vi "SMC TestProgram.vi"() -> ()   [LabVIEW 2015]
uses:
  SubVIs/JS_Misc.llb/JS_Axis_PM.ctl
  SubVIs/JS_Comm.llb/Comm_Paras.ctl
  SubVIs/JS_Comm.llb/Comm_Method.ctl
  SMC SubVIs/SMC_SubVIs.llb/SMC Paras.ctl
  SMC SubVIs/SMC_SubVIs.llb/VENUSNr.ctl
  SMC SubVIs/SMC_SubVIs.llb/glb_stop.vi
  SMC SubVIs/SMC_SubVIs.llb/glb_pos.vi
panel:
  in  "Show Dialog Box":bool=TRUE
  in  "Error":bool
  in  "Controller Nr":u8=3 min=1 max=10 step=1
  out "Communication":bool
  out "Communication Error":bool
  out "Position":dbl[](array[numeric]) format="%.6f"
  out "Moving":bool
  in  "Stop":bool
  in  "Tab Control":enum32{"Standard", "low level"}(tab)
  in  "Velocity":bool
  in  "Move absolute":bool
  in  "Destination [mm]":dbl[](array[numeric]) format="%.6f"
  in  "Manual Control":T1[](array[typedef])
  in  "RefMove":bool
  in  "SetZero":bool
  in  "StepWidth [mm]":dbl=1.0 format="%.6f"
  in  "RangeMeasure":bool
  in  "Calibrate":bool
  in  "Switch Status":bool
  in  "Limit":bool
  in  "Maeander":bool
  in  "Sequence":bool
  in  "Get Error":bool
  out "ErrorText":string
  out "Error Code":string
  out "Result":string
  in  "Command":string
  in  "Send":bool
  out "End Prog":bool
  out "error out":errorcluster
  in  "End Program":bool
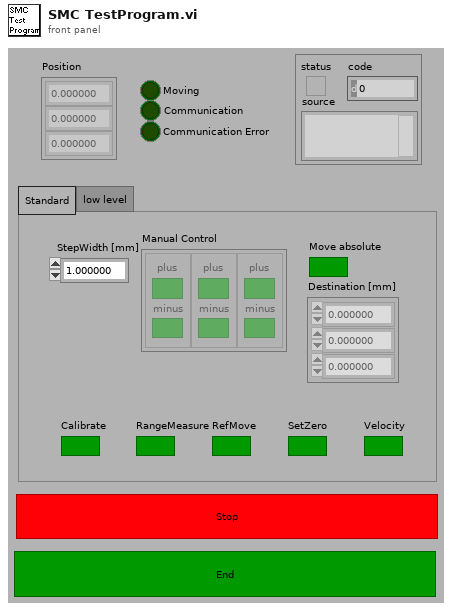
[diagram p1: front panel]
types:
  T1 = typedef "JS_Axis_PM.ctl" = cluster{"minus":bool, "plus":bool}
  T2 = typedef "SMC Paras.ctl" = cluster{"VENUS Language":T3, "Number of Axis":u8, "Controller Nr":u8, "Simulation":bool}
  T3 = typedef "VENUSNr.ctl" = enum16{"VENUS 2", "VENUS 1"}
  T4 = typedef "Comm_Paras.ctl" = cluster{"Comm Method":T5, "Com Port":i32, "Baud Rate":u32, "IP Address":string, "Remote Port":u16, "GPIB Address":string, "VISA Resource Name":refnum<visa-resource-name>, "Visa Baud Rate":u32, "Visa Serial":bool}
  T5 = typedef "Comm_Method.ctl" = enum16{"RS232", "TCPIP", "GPIB", "VISA"}
  T6 = typedef "Sequence Paras.ctl" = cluster{"Number of cycles":i32, "Start position":dbl[], "End position":dbl[]}
  T7 = typedef "Maeander_Paras.ctl" = cluster{"Number":i32, "X Start":dbl, "Y Start":dbl, "X Size":dbl, "Y Size":dbl}
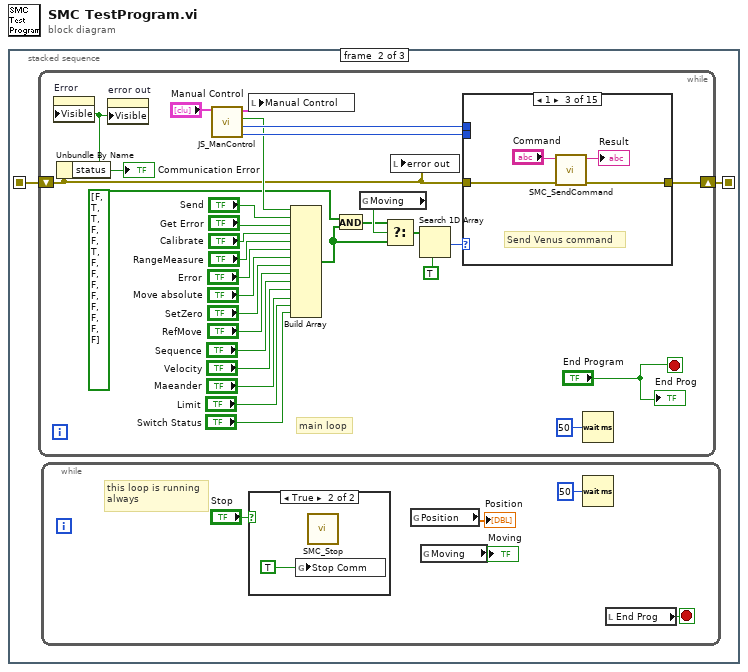
[diagram p0: block diagram]
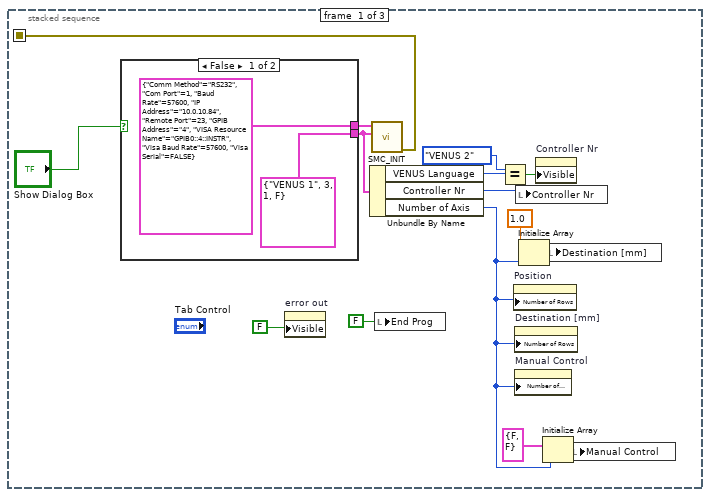
[diagram p2: hidden frame]
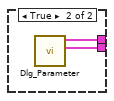
[diagram p3: hidden frame]
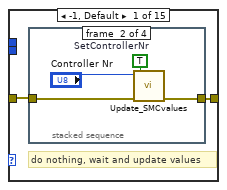
[diagram p5: hidden frame]
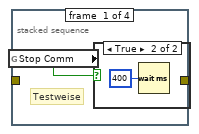
[diagram p6: hidden frame]
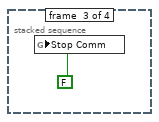
[diagram p8: hidden frame]
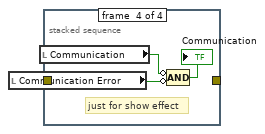
[diagram p9: hidden frame]
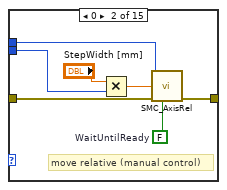
[diagram p10: hidden frame]
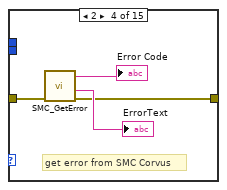
[diagram p11: hidden frame]
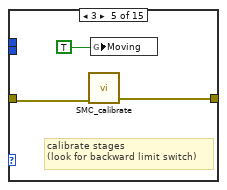
[diagram p12: hidden frame]
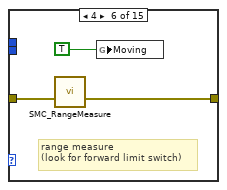
[diagram p13: hidden frame]
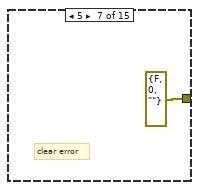
[diagram p14: hidden frame]
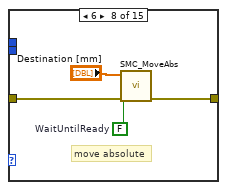
[diagram p15: hidden frame]
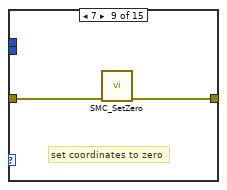
[diagram p16: hidden frame]
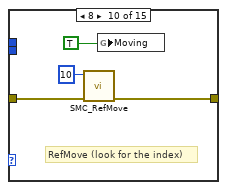
[diagram p17: hidden frame]
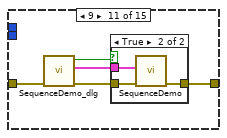
[diagram p18: hidden frame]
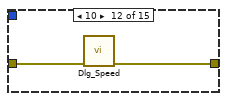
[diagram p20: hidden frame]
diagram:
  n1 = stacked-sequence {
    seq-local: [w11 _ _] -> [_ w21 _]
    seq-local: [_ w20 _] -> [_ _ w128]
    frame #0 {
      n2 = case shown="False" "Show Dialog Box" {
        tunnel: [T4 {"Comm Method"=enum."RS232", "Com Port"=1, "Baud Rate"=57600, "IP Address"="10.0.10.84", "Remote Port"=23, "GPIB Address"="4", "VISA Resource Name"="GPIB0::4::INSTR", "Visa Baud Rate"=57600, "Visa Serial"=FALSE} ("Communication Parameter") w19] -> w9
        tunnel: [T2 {"VENUS Language"=enum."VENUS 1", "Number of Axis"=3, "Controller Nr"=1, "Simulation"=FALSE} ("SMC Parameter") w18] -> w7
        frame False {
        }
        frame True {
          n3 = call "Dlg_Parameter.vi"() -> ("SMC Parameter"=w18:T2, "Communication Parameter"=w19:T4)  [unwired: 10 in]
        }
      }
      n4 = property on="error out" class="Clust (strict)"("Visible"=FALSE ("Write Attribute")) -> ()  [unwired: 2 in, 2 out]
      n5 = Unbundle By Name(w7) -> ("VENUS Language"=w6:T3, "Controller Nr"=w4:u8, "Number of Axis"=w2:u8)
      n6 = call "SMC_INIT.vi"("SMC Parameter"=w7, "Communication Parameter"=w9) -> ("error out"=w11:errorcluster)  [unwired: 9 in]
      n7 = local write "End Prog"(FALSE ("End Prog")) -> ()
      n8 = Equal?(x=enum16{"VENUS 2", "VENUS 1"}."VENUS 2" ("y"), y=w6) -> (x = y?=w8:bool)
      n9 = property on="Position" class="Arr (strict)"("Number of Rows"=w2) -> ()  [unwired: 2 in, 2 out]
      n10 = property on="Destination [mm]" class="Arr (strict)"("Number of Rows"=w2) -> ()  [unwired: 2 in, 2 out]
      n11 = property on="Manual Control" class="Arr"("Number of Columns"=w2) -> ()  [unwired: 2 in, 2 out]
      n12 = local write "Controller Nr"(w4) -> ()
      n13 = Initialize Array(1.0, w2) -> (w12:dbl[])
      n14 = property on="Controller Nr" class="DigNum (strict)"("Visible"=w8) -> ()  [unwired: 2 in, 2 out]
      n15 = Initialize Array(T1 {"minus"=FALSE, "plus"=FALSE} ("Cluster"), w2) -> (w1:T1[])
      n16 = local write "Destination [mm]"(w12) -> ()
      n17 = local write "Manual Control"(w1) -> ()
    }
    frame #1 {
      n18 = while {
        shift-right: [w30] -> w20
        shift-left: w21 -> [w28]
        stop <- "End Program" stop-if-true
        # "main loop"
        n19 = Unbundle By Name(w28) -> ("status"=w29:bool)
        "Communication Error" <- w29
        n20 = property on="Error" class="Bool"("Visible"=w29) -> ()  [unwired: 2 in, 2 out]
        n21 = property on="error out" class="Clust (strict)"("Visible"=w29) -> ()  [unwired: 2 in, 2 out]
        n22 = call "JS_ManControl.vi"("Manual Control in"="Manual Control") -> ("Manual Control out"=w47:T1[], "Fire"=w45:bool, "AxisNr"=w48:i32, "sign"=w46:i8)
        n23 = local write "Manual Control"(w47) -> ()
        n24 = Build Array(w45, "Send", "Get Error", "Calibrate", "RangeMeasure", "Error", "Move absolute", "SetZero", "RefMove", "Sequence", "Velocity", "Maeander", "Limit", "Switch Status") -> (w37:bool[])
        n25 = And(x=bool[] [FALSE, TRUE, TRUE, FALSE, FALSE, TRUE, FALSE, FALSE, FALSE, FALSE, FALSE, FALSE, FALSE, FALSE] ("Array Constant"), y=w37) -> (x .and. y?=w36:bool[])
        n26 = global read "glb_pos.vi" "Moving"() -> (w39:bool)
        n27 = Select(t=w36, s=w39, f=w37) -> (s? t:f=w40:bool[])
        n28 = local write "error out"(w28) -> ()
        n29 = Search 1D Array(1D array=w40, element=TRUE) -> (index of element=w54:i32)  [unwired: 1 in]
        n30 = case shown="1" w54 {
          tunnel: w28 -> [w58 w76 w80 w82 w87 w90 _ w95 w97 w101 w105 w112 w117 w123 w125]
          tunnel: [w59 w75 w79 w81 w86 w89 errorcluster {"status"=FALSE, "code"=0, "source"=""} ("error out") w94 w96 w100 w106 w111 w115 w122 w124] -> w30
          tunnel: w48 -> [_ w71 _ _ _ _ _ _ _ _ _ _ _ _ _]
          tunnel: w46 -> [_ w74 _ _ _ _ _ _ _ _ _ _ _ _ _]
          frame -1, Default {
            # "do nothing, wait and update values"
            n31 = stacked-sequence {
              tunnel: [_ w65 _ _] -> w59
              tunnel: w58 -> [_ w64 _ _]
              frame #0 {
                # "Testweise"
                n32 = global read "glb_stop.vi" "Stop Comm"() -> (w60:bool)
                n33 = case shown="True" w60 {
                  frame False {
                  }
                  frame True {
                    n34 = Wait (ms)(milliseconds to wait=u32 400) -> ()  [unwired: 1 out]
                  }
                }
              }
              frame #1 {
                w62 = TRUE  # SetControllerNr
                n35 = call "Update_SMCvalues.vi"("error in"=w64, "SetControllerNr"=w62, "Controller Nr"="Controller Nr") -> ("error out"=w65:errorcluster)  [unwired: 7 in, 1 out]
              }
              frame #2 {
                n36 = global write "glb_stop.vi" "Stop Comm"(FALSE ("Stop Comm")) -> ()
              }
              frame #3 {
                # "just for show effect"
                n37 = local read "Communication Error"() -> (w67:bool)
                n38 = local read "Communication"() -> (w68:bool)
                n39 = Compound Arithmetic op=AND(invert w68, invert w67) -> (→"Communication":bool)
              }
            }
          }
          frame 0 {
            w70 = FALSE  # WaitUntilReady
            # "move relative (manual control)"
            n40 = Multiply(x="StepWidth [mm]", y=w74) -> (x*y=w73:dbl)
            n41 = call "SMC_AxisRel.vi"("error in (no error)"=w76, "WaitUntilReady"=w70, "Distance"=w73, "AxisNr"=w71) -> ("error out"=w75:errorcluster)  [unwired: 7 in]
          }
          frame 1 {
            # "Send Venus command"
            n42 = call "SMC_SendCommand.vi"("error in (no error)"=w80, "Command"="Command") -> ("error out"=w79:errorcluster, "Answer"=→"Result":string)  [unwired: 8 in]
          }
          frame 2 {
            # "get error from SMC Corvus"
            n43 = call "SMC_GetError.vi"("error in (no error)"=w82) -> ("error out"=w81:errorcluster, "ErrorText"=→"ErrorText":string, "Answer"=→"Error Code":string)  [unwired: 8 in]
          }
          frame 3 {
            # "calibrate stages\n(look for backward limit switch)"
            n44 = call "SMC_calibrate.vi"("error in (no error)"=w87) -> ("error out"=w86:errorcluster)  [unwired: 10 in]
            n45 = global write "glb_pos.vi" "Moving"(TRUE ("Moving")) -> ()
          }
          frame 4 {
            # "range measure\n(look for forward limit switch)"
            n46 = call "SMC_RangeMeasure.vi"("error in (no error)"=w90) -> ("error out"=w89:errorcluster)  [unwired: 10 in]
            n47 = global write "glb_pos.vi" "Moving"(TRUE ("Moving")) -> ()
          }
          frame 5 {
            # "clear error"
          }
          frame 6 {
            w92 = FALSE  # WaitUntilReady
            # "move absolute"
            n48 = call "SMC_MoveAbs.vi"("error in (no error)"=w95, "WaitUntilReady"=w92, "Input Array"="Destination [mm]") -> ("error out"=w94:errorcluster)  [unwired: 8 in]
          }
          frame 7 {
            # "set coordinates to zero"
            n49 = call "SMC_SetZero.vi"("error in (no error)"=w97) -> ("error out"=w96:errorcluster)  [unwired: 10 in]
          }
          frame 8 {
            # "RefMove (look for the index)"
            n50 = call "SMC_RefMove.vi"("error in (no error)"=w101, "Number of revolutions"=u8 10) -> ("error out"=w100:errorcluster)  [unwired: 9 in]
            n51 = global write "glb_pos.vi" "Moving"(TRUE ("Moving")) -> ()
          }
          frame 9 {
            n52 = call "SequenceDemo_dlg.vi"("error in (no error)"=w105) -> ("error out"=w104:errorcluster, "Sequence Paras"=w102:T6, "OK Out"=w103:bool)  [unwired: 8 in]
            n53 = case shown="True" w103 {
              tunnel: w104 -> [w107 w110]
              tunnel: [w107 w109] -> w106
              tunnel: w102 -> [_ w108]
              frame False {
              }
              frame True {
                n54 = call "SequenceDemo.vi"("error in (no error)"=w110, "Sequence Paras"=w108) -> ("error out"=w109:errorcluster)  [unwired: 9 in]
              }
            }
          }
          frame 10 {
            n55 = call "Dlg_Speed.vi"("error in (no error)"=w112) -> ("error out"=w111:errorcluster)  [unwired: 10 in]
          }
          frame 11 {
            n56 = call "MaeanderDemo_Dlg.vi"("error in (no error)"=w117) -> ("error out"=w116:errorcluster, "Maeander Parameter"=w113:T7, "OK Out"=w114:bool)  [unwired: 8 in]
            n57 = case shown="True" w114 {
              tunnel: w116 -> [w118 w121]
              tunnel: [w118 w120] -> w115
              tunnel: w113 -> [_ w119]
              frame False {
              }
              frame True {
                n58 = call "MaeanderDemo.vi"("error in (no error)"=w121, "Maeander Parameter"=w119) -> ("error out"=w120:errorcluster)  [unwired: 9 in]
              }
            }
          }
          frame 12 {
            n59 = call "SMC_GetLimit.vi"("error in (no error)"=w123) -> ("error out"=w122:errorcluster)  [unwired: 8 in, 2 out]
          }
          frame 13 {
            n60 = call "SMC_GetSwSt.vi"("error in (no error)"=w125) -> ("error out"=w124:errorcluster)  [unwired: 8 in, 2 out]
          }
        }
        n61 = Wait (ms)(milliseconds to wait=u32 50) -> ()  [unwired: 1 out]
        "End Prog" <- "End Program"
      }
      n62 = while {
        stop <- w24 stop-if-true
        # "this loop is running\nalways"
        n63 = case shown="True" "Stop" {
          frame False {
          }
          frame True {
            n64 = global write "glb_stop.vi" "Stop Comm"(TRUE ("Stop Comm")) -> ()
            n65 = call "SMC_Stop.vi"() -> ()  [unwired: 11 in, 1 out]
          }
        }
        n66 = global read "glb_pos.vi" "Position"() -> (→"Position":dbl[])
        n67 = global read "glb_pos.vi" "Moving"() -> (→"Moving":bool)
        n68 = Wait (ms)(milliseconds to wait=u32 50) -> ()  [unwired: 1 out]
        n69 = local read "End Prog"() -> (w24:bool)
      }
    }
    frame #2 {
      n70 = call "SMC_Close.vi"("error in (no error)"=w128) -> ("error out"=→"error out":errorcluster)  [unwired: 10 in]
      n71 = property on="Controller Nr" class="DigNum (strict)"("Visible"=FALSE) -> ()  [unwired: 2 in, 2 out]
      n72 = property on="error out" class="Clust (strict)"("Visible"=TRUE ("Write Attribute")) -> ()  [unwired: 2 in, 2 out]
    }
  }
